vi "ADI_IMU_ADIS16448_HardwareResetDelay.vi"(7 "Delay (ms)":u32=200, 8 "error in":errorcluster) -> (0 "error out":errorcluster)   [LabVIEW 2016, in "ADIS16448_IMU.lvlib"]
uses:
  ADIS16448_IMU.lvlib
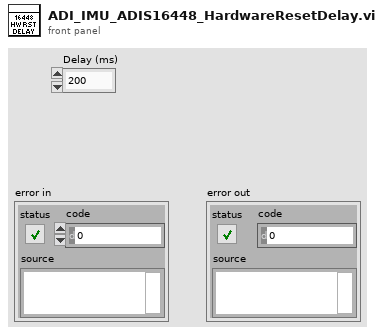
[diagram p1: front panel]
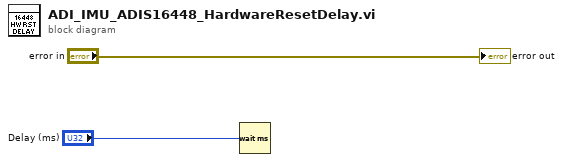
[diagram p0: block diagram]
diagram:
  n1 = Wait (ms)(milliseconds to wait="Delay (ms)") -> ()  [unwired: 1 out]
  "error out" <- "error in"
